vi "GetMonitorChannelValue.vi"(8 "error in":errorcluster, 10 "Channel number (1-24)":i32=1 min=1 max=24 step=1, 11 "VISA resource name":refnum<visa-resource-name>) -> (0 "error out":errorcluster, 1 "Monitor channel value":sgl format="%0.3f", 2 "Monitor Channel Value String":string, 3 "VISA resource name out":refnum<visa-resource-name>)   [LabVIEW 2023, in "Thermotron 8800.lvlib"]
doc: "MNTR\nCommand name: Send monitor channel value\nCommand type: Variable\nDescription: Queries the 8800 for the current value of the selected monitor channel.\nSyntax: MNTRn?\nWhere n is the monitor channel number (1 through 24).\nData type: Decimal\nQuery example: MNTR1?\n8800 response: -35.8 (The current value of monitor channel 1 is -35.8.)"
uses:
  Thermotron 8800.lvlib
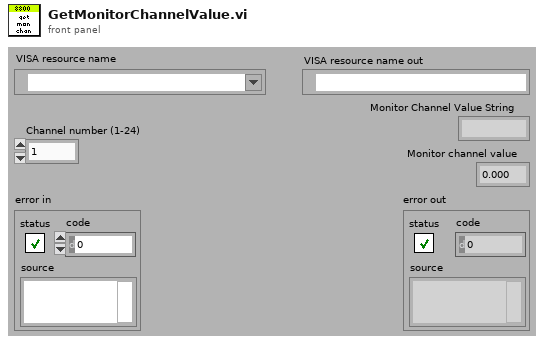
[diagram p1: front panel]
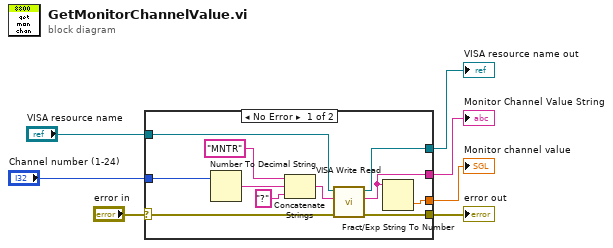
[diagram p0: block diagram]
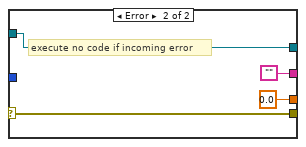
[diagram p2: hidden frame]
diagram:
  n1 = case shown="No Error" "error in" {
    selector: "error in" -> [w16 w21]
    tunnel: [w13 w21] -> w6
    tunnel: [w14 w22] -> w5
    tunnel: "VISA resource name" -> [w15 w22]
    tunnel: [w12 ""] -> w3
    tunnel: [w11 sgl 0.0] -> w2
    tunnel: "Channel number (1-24)" -> [w8 _]
    frame No Error {
      n2 = Number To Decimal String(number=w8) -> (decimal integer string=w9:string)  [unwired: 1 in]
      n3 = Concatenate Strings("MNTR" ("8800 Command"), w9, "?" ("8800 Command")) -> (w18:string)
      n4 = call "VISA Write Read.vi"("error in (no error)"=w16, "8800 Command"=w18, "VISA Refnum in"=w15) -> ("error out"=w13:errorcluster, "read buffer"=w12:string, "VISA Refnum out"=w14:refnum<visa-resource-name>)  [unwired: 6 in]
      n5 = Fract/Exp String To Number(string=w12) -> (number=w11:dbl)  [unwired: 3 in, 1 out]
    }
    frame Error {
      # "execute no code if incoming error"
    }
  }
  "VISA resource name out" <- w5
  "error out" <- w6
  "Monitor Channel Value String" <- w3
  "Monitor channel value" <- w2
